vi "3D02_Grab_and_Attributes_Setup.vi"() -> ()   [LabVIEW 2012]
doc: "The Grab and Attributes Setup example VI allows the user to view the current attributes and settings, update attribute settings, acquire images continuously, and display the images in an image control."
uses:
  <vilib>/userDefined/High Color/IMAQdx.ctl
  <vilib>/vision/driver/IMAQdx.llb/IMAQdx Acquisition Mode.ctl
  <vilib>/vision/driver/IMAQdx.llb/IMAQdx Buffer Number Mode.ctl
  <vilib>/vision/driver/NI_Vision_Acquisition_Software.lvlib
  <resource>/objmgr/imaqdx.rc
  <userlib>/Photonfocus Toolkit/Photonfocus_Toolkit.lvlib
panel:
  out "MissedFrameCombineTriggerCounter":u8[](array[numeric])
  out "MissedBurstTriggerCounter":u8[](array[numeric])
  out "MissedTriggerCounter":u8[](array[numeric])
  out "EncoderPosition":u32[](array[numeric])
  out "RealTimeCounter":u32[](array[numeric])
  out "ImageCounter":u32[](array[numeric])
  out "Quality":u8[][](graph)
  out "Width":u8[][](graph)
  out "Peak":sgl[][](graph)
  out "FrameCombine_NrOfFrames":u32
  out "FrameCombine_Enable":bool
  out "PeakDetector_Mode":u32
  in  "Grab":bool
  out "Tooltip":string
  out "Units":string
  out "Tab Control Ref":T1
  in  "Tab Control":T2(tab)
  in  "U32 Value Control":u32(slide) scale=4.0..4044.0
  in  "DBL Value Control":dbl(slide) min=1.0 max=1028.0 step=1.0 scale=1.0..1028.0
  in  "String Value Control":string
  in  "Enum Value Control":u32(ring) items=["Mode_2Donly", "Mode_2Dand3D", "Mode_3Donly"]
  in  "Boolean Value Control":bool=TRUE
  in  "Command Value Control":bool
  in  "Attribute Table":string(tree)
  out "Frame Rate":dbl(knob) scale=0.0..100.0 scale format="%.1f"
  out "Image":T3(plugin-control)
  out "Buffer Number":u32
  in  "Camera Name":T4
  in  "stop":bool
  # "3D Data"
  # "Status info"
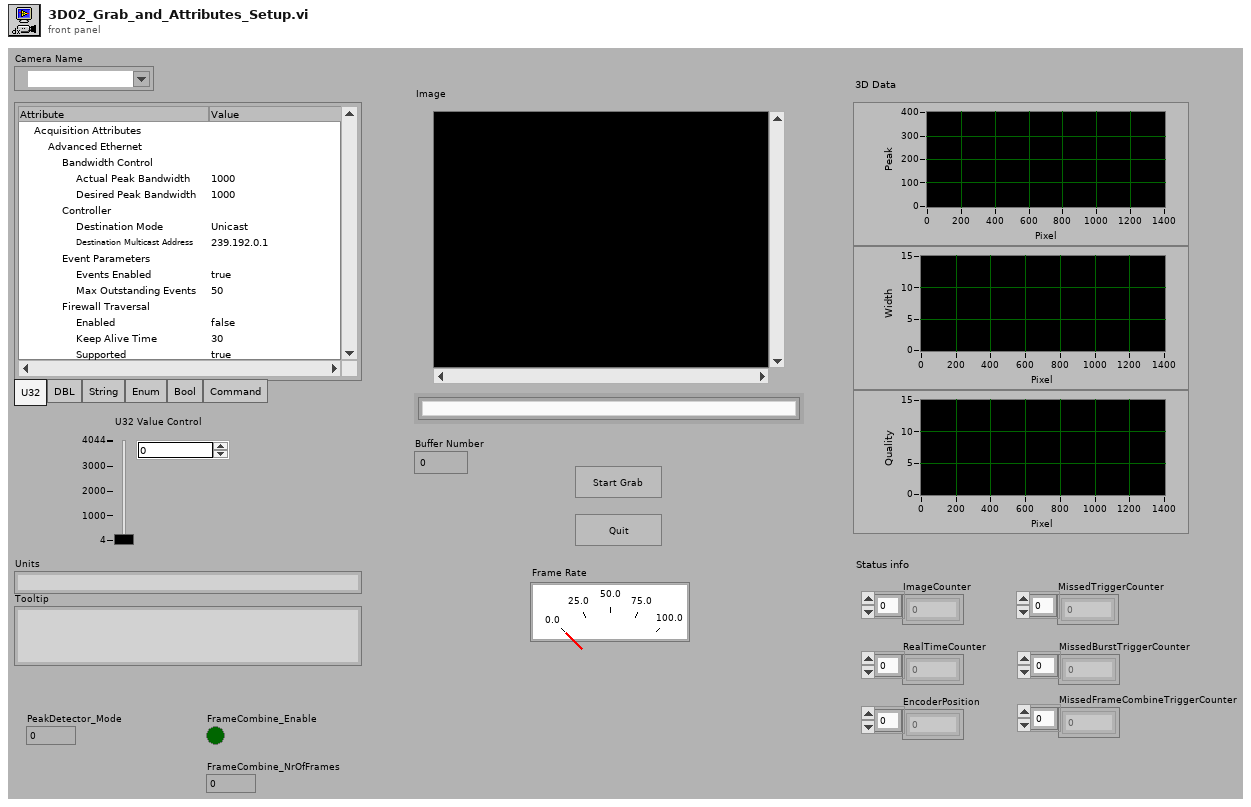
[diagram p1: front panel]
types:
  T1 = cluster{"Tab Control":refnum<vi>, "U32 Value Control":refnum<vi>, "DBL Value Control":refnum<vi>, "String Value Control":refnum<vi>, "Enum Value Control":refnum<vi>, "Boolean Value Control":refnum<vi>, "Command Value Control":refnum<vi>}
  T2 = enum32{"U32", "DBL", "String", "Enum", "Bool", "Command"}
  T3 = typedef "IMAQ Image.ctl" = refnum<image>
  T4 = typedef "IMAQdx.ctl" = refnum<k21>
  T5 = typedef "NI_Vision_Acquisition_Software.lvlib/IMAQdx Acquisition Mode.ctl" = enum32{"One Shot", "Continuous"}
  T6 = typedef "NI_Vision_Acquisition_Software.lvlib/IMAQdx Buffer Number Mode.ctl" = enum32{"Next", "Last", "Buffer Number"}
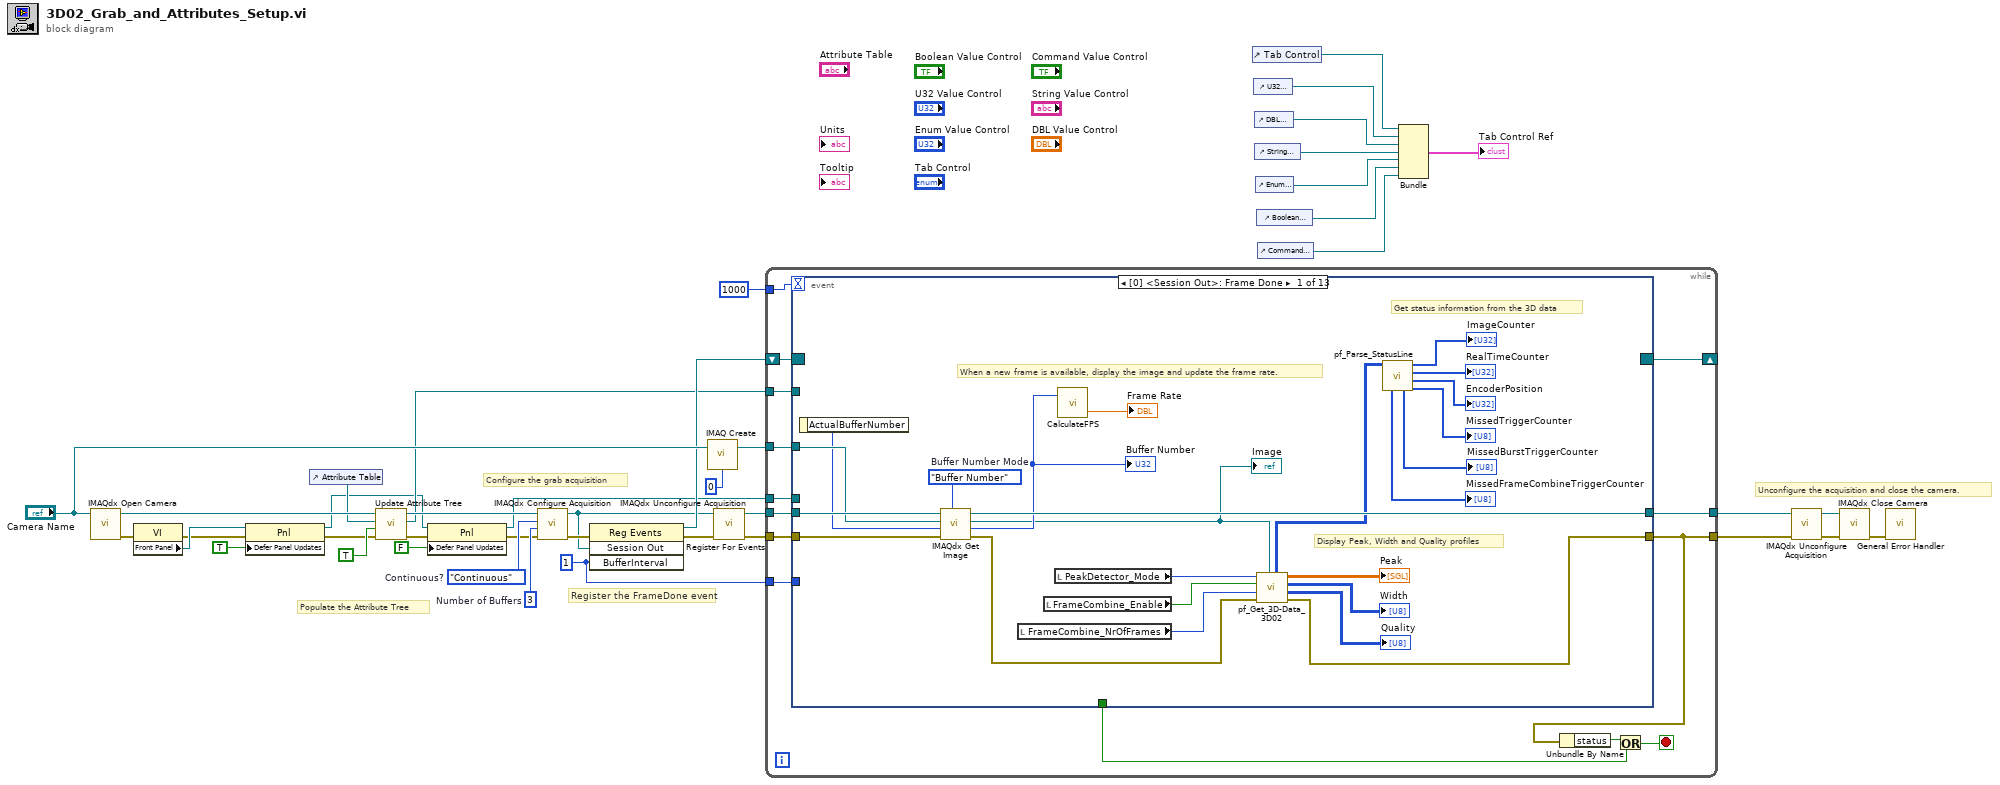
[diagram p0: block diagram]
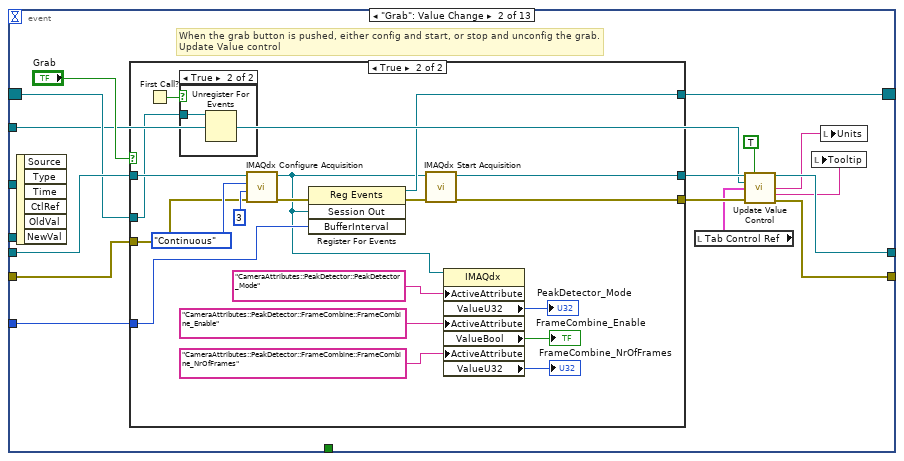
[diagram p2: hidden frame]
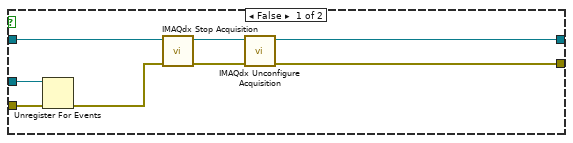
[diagram p3: hidden frame]
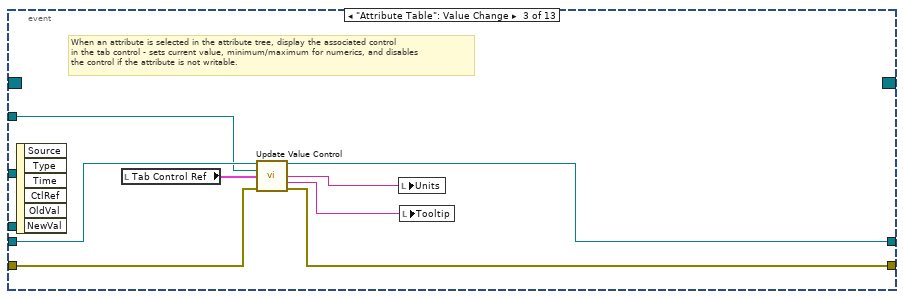
[diagram p5: hidden frame]
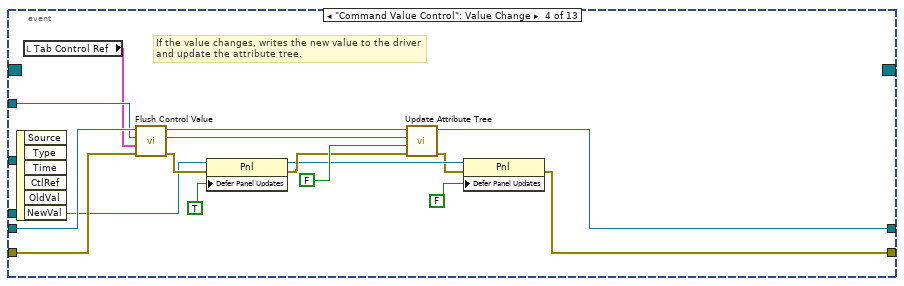
[diagram p6: hidden frame]
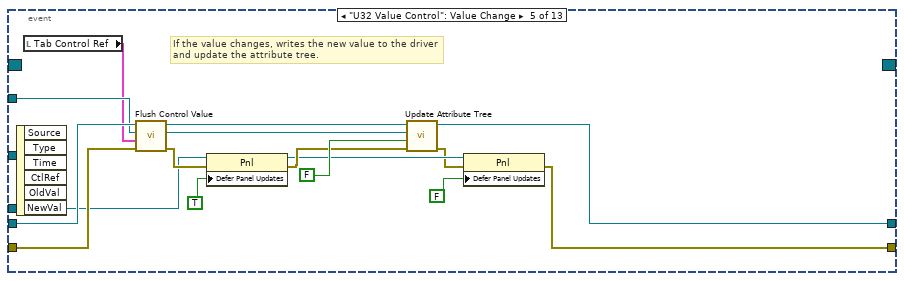
[diagram p7: hidden frame]
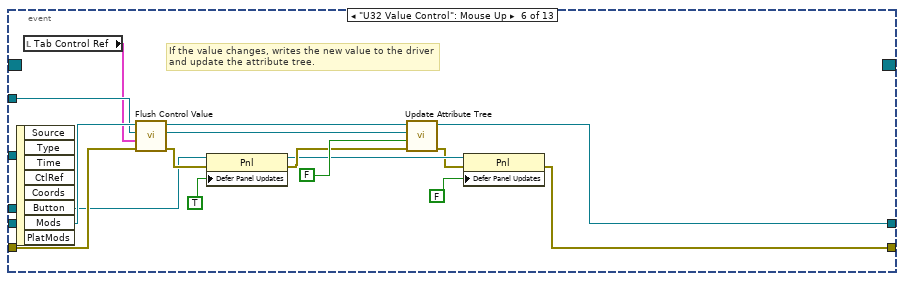
[diagram p8: hidden frame]
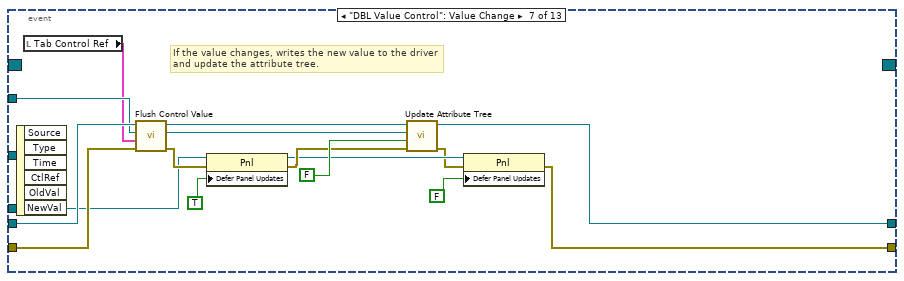
[diagram p9: hidden frame]
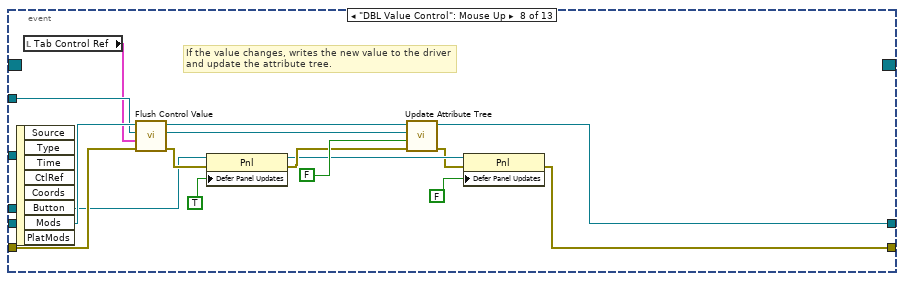
[diagram p10: hidden frame]
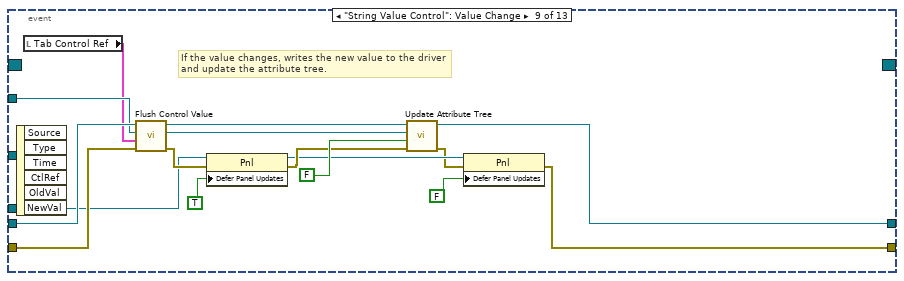
[diagram p11: hidden frame]
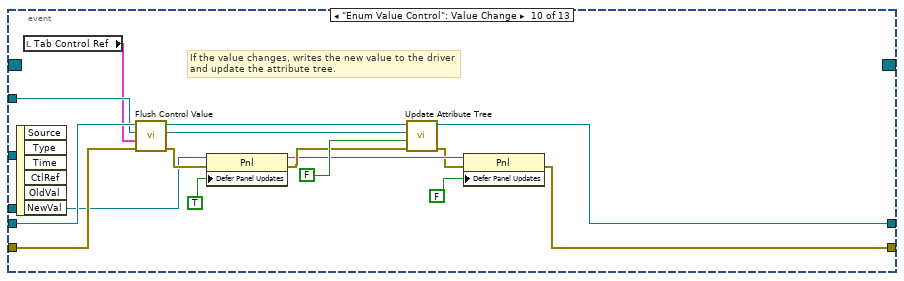
[diagram p12: hidden frame]
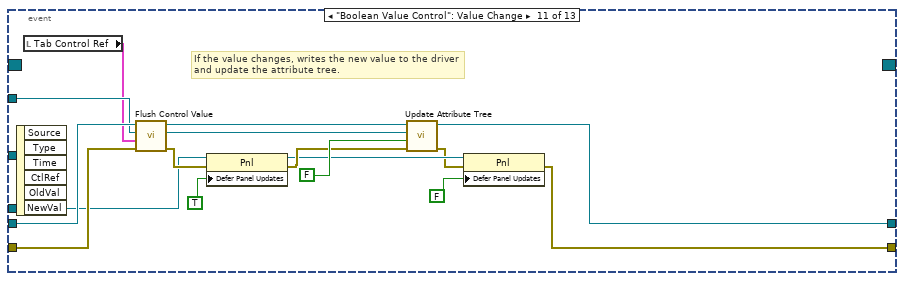
[diagram p13: hidden frame]
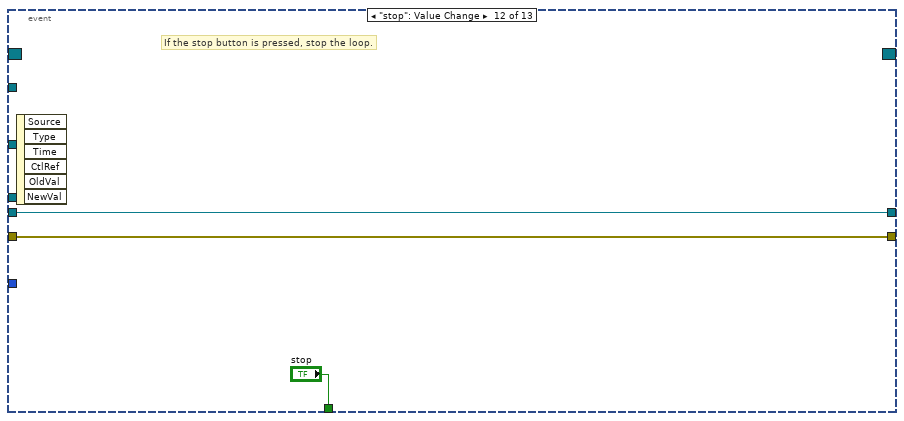
[diagram p14: hidden frame]
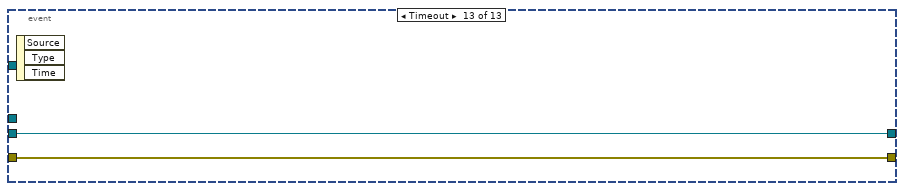
[diagram p15: hidden frame]
diagram:
  w6 = u32 1 ("BufferInterval")
  w37 = u32 3  # Number of Buffers
  w38 = IMAQdx_Acquisition_Mode."Continuous"  # Continuous?
  # "Unconfigure the acquisition and close the camera."
  # "Register the FrameDone event"
  # "Configure the grab acquisition"
  # "Populate the Attribute Tree"
  n1 = call <vilib>:"IMAQdx Open Camera.vi"("Session In"="Camera Name") -> ("error out"=w9:errorcluster, "Session Out"=w23:T4)  [unwired: 2 in, 7 out]
  n2 = property class="VI"(error in=w9) -> (error out=w10:errorcluster, "Front Panel"=w11:refnum<vi>)  [unwired: 1 in, 1 out]
  n3 = property class="Pnl"(reference=w11, error in=w10, "Defer Panel Updates"=TRUE) -> (reference out=w14:refnum<vi>, error out=w18:errorcluster)
  n4 = control-ref of="Attribute Table"() -> (w21:refnum<vi>)
  n5 = call <userlib>:"Update Attribute Tree.vi"("error in"=w18, "Flush Tree?"=TRUE, "Tree Control In"=w21, "Camera Name In"=w23) -> ("error out"=w17:errorcluster, "Tree Control Out"=w19:refnum<vi>, "Session Out"=w22:T4)  [unwired: 1 out]
  n6 = property class="Pnl"(reference=w14, error in=w17, "Defer Panel Updates"=FALSE) -> (reference out=w13:refnum<vi>, error out=w15:errorcluster)
  n7 = call <vilib>:"IMAQdx Configure Acquisition.vi"("error in"=w15, "Number of Buffers"=w37, "Continuous?"=w38, "Session In"=w22) -> ("error out"=w34:errorcluster, "Session Out"=w3:T4)  [unwired: 6 out]
  n8 = register-events(error in=w34, w3, w6) -> (reference out=w33:refnum<event-registration>, error out=w5:errorcluster)  [unwired: 1 in]
  n9 = call "IMAQ Create"("Image Name"="Camera Name", "Image Type"=0) -> ("New Image"=w41:T3)  [unwired: 2 in, 2 out]
  n10 = call <vilib>:"IMAQdx Unconfigure Acquisition.vi"("error in"=w5, "Session In"=w3) -> ("error out"=w4:errorcluster, "Session Out"=w2:T4)  [unwired: 8 out]
  n11 = while {
    tunnel: [w50] -> w8
    tunnel: w4 -> [w52]
    tunnel: w2 -> [w53]
    tunnel: [w49] -> w7
    tunnel: w41 -> [w51]
    tunnel: 1000 -> [w47]
    tunnel: w19 -> [w46]
    tunnel: w13 -> [w45]
    tunnel: w6 -> [w43]
    shift-right: [w42] -> _
    shift-left: w33 -> [w48]
    stop <- w55 stop-if-true
    n12 = event shown="[0] <Session Out>: Frame Done" {
      selector: w48 -> [_ w91 _ _ _ _ _ _ _ _ _ _ _]
      dyn-events: [_ w92 _ _ _ _ _ _ _ _ _ _ _] -> w42
      timeout: w47 -> [_ _ _ _ _ _ _ _ _ _ _ _ _]
      tunnel: w53 -> [w79 w94 w130 w145 w161 w177 w193 w209 w225 w241 w257 w260 w262]
      tunnel: w52 -> [w78 w90 w128 w146 w162 w178 w194 w210 w226 w242 w258 w259 w263]
      tunnel: w51 -> [w77 _ _ _ _ _ _ _ _ _ _ _ _]
      tunnel: [w76 w88 w129 w131 w147 w163 w179 w195 w211 w227 w243 w260 w262] -> w50
      tunnel: [w68 w86 w127 w132 w148 w164 w180 w196 w212 w228 w244 w259 w263] -> w49
      tunnel: w46 -> [_ w84 w123 w143 w159 w175 w191 w207 w223 w239 w255 _ _]
      tunnel: w45 -> [_ _ _ w137 w153 w169 w185 w201 w217 w233 w249 _ _]
      tunnel: [_ _ _ _ _ _ _ _ _ _ _ "stop" _] -> w44
      tunnel: w43 -> [_ w80 _ _ _ _ _ _ _ _ _ _ _]
      event event #0x0 {
        w74 = IMAQdx_Buffer_Number_Mode."Buffer Number"  # Buffer Number Mode
        # "Get status information from the 3D data"
        # "Display Peak, Width and Quality profiles"
        # "When a new frame is available, display the image and update the frame rate."
        n13 = event-data() -> ("ActualBufferNumber"=w73:u32)  [unwired: 1 out]
        n14 = call <vilib>:"IMAQdx Get Image.vi"("Buffer Number Mode (Next)"=w74, "error in"=w78, "Buffer Number In"=w73, "Image In"=w77, "Session In"=w79) -> ("error out"=w69:errorcluster, "Buffer Number Out"=w72:u32, "Image Out"=w70:T3, "Session Out"=w76:T4)  [unwired: 3 out]
        "Image" <- w70
        "Buffer Number" <- w72
        n15 = local read "FrameCombine_NrOfFrames"() -> (w63:u32)
        n16 = local read "FrameCombine_Enable"() -> (w64:bool)
        n17 = local read "PeakDetector_Mode"() -> (w71:u32)
        n18 = call <userlib>:"CalculateFPS.vi"("buffer number"=w72) -> ("processed FPS"=→"Frame Rate":dbl)  [unwired: 2 out]
        n19 = call <userlib>:"pf_Get_3D-Data_3D02.vi"("Aquired Image"=w70, "error in (no error)"=w69, "FrameCombine_NrOfFrames"=w63, "FrameCombine_Enable"=w64, "PealDetector_Mode"=w71) -> ("error out"=w68:errorcluster, "Quality Profile"=→"Quality":u8[][], "Width Profile"=→"Width":u8[][], "Peak Profile"=→"Peak":sgl[][], "Status Line"=w56:u8[][])  [unwired: 2 in]
        n20 = call <userlib>:"pf_Parse_StatusLine.vi"("Status Line"=w56) -> ("MissedTriggerCounter"=→"MissedTriggerCounter":u8[], "EncoderPosition"=→"EncoderPosition":u32[], "RealTimeCounter"=→"RealTimeCounter":u32[], "ImageCounter"=→"ImageCounter":u32[], "MissedBurstTriggerCounter"=→"MissedBurstTriggerCounter":u8[], "MissedFrameCombineTriggerCounter"=→"MissedFrameCombineTriggerCounter":u8[])  [unwired: 5 in]
      }
      event "Grab": Value Change {
        # "When the grab button is pushed, either config and start, or stop and unconfig the grab.\nUpdate Value control"
        n21 = event-data() -> ()  [unwired: 7 out]
        n22 = case shown="True" "Grab" {
          tunnel: w94 -> [w102 w119]
          tunnel: [w99 w121] -> w89
          tunnel: [w98 w120] -> w87
          tunnel: [_ w114] -> w92
          tunnel: w80 -> [_ w110]
          tunnel: w91 -> [w97 w112]
          tunnel: w90 -> [w95 w113]
          frame False {
            n23 = Unregister For Events(event registration refnum=w97, error in=w95) -> (error out=w96:errorcluster)
            n24 = call <vilib>:"IMAQdx Stop Acquisition.vi"("error in"=w96, "Session In"=w102) -> ("error out"=w100:errorcluster, "Session Out"=w101:T4)  [unwired: 8 out]
            n25 = call <vilib>:"IMAQdx Unconfigure Acquisition.vi"("error in"=w100, "Session In"=w101) -> ("error out"=w98:errorcluster, "Session Out"=w99:T4)  [unwired: 8 out]
          }
          frame True {
            n26 = First Call?() -> (First Call?: T/F=w111:bool)
            n27 = case shown="True" w111 {
              tunnel: w112 -> [_ w122]
              frame False {
              }
              frame True {
                n28 = Unregister For Events(event registration refnum=w122) -> ()  [unwired: 1 in, 1 out]
              }
            }
            n29 = call <vilib>:"IMAQdx Configure Acquisition.vi"("error in"=w113, "Number of Buffers"=u32 3, "Continuous?"=IMAQdx_Acquisition_Mode."Continuous", "Session In"=w119) -> ("error out"=w116:errorcluster, "Session Out"=w104:T4)  [unwired: 6 out]
            n30 = register-events(error in=w116, w104, w110) -> (reference out=w114:refnum<event-registration>, error out=w115:errorcluster)  [unwired: 1 in]
            n31 = call <vilib>:"IMAQdx Start Acquisition.vi"("error in"=w115, "Session In"=w104) -> ("error out"=w120:errorcluster, "Session Out"=w121:T4)  [unwired: 8 out]
            n32 = property class="IMAQdx"(reference=w104, "ActiveAttribute"="CameraAttributes::PeakDetector::PeakDetector_Mode", "ActiveAttribute"="CameraAttributes::PeakDetector::FrameCombine::FrameCombine_Enable", "ActiveAttribute"="CameraAttributes::PeakDetector::FrameCombine::FrameCombine_NrOfFrames") -> ("ValueU32"=→"PeakDetector_Mode":u32, "ValueBool"=→"FrameCombine_Enable":bool, "ValueU32"=→"FrameCombine_NrOfFrames":u32)  [unwired: 1 in, 2 out]
          }
        }
        n33 = local read "Tab Control Ref"() -> (w85:T1)
        n34 = call <userlib>:"Update Value Control.vi"("Session In"=w89, "Force update?"=TRUE, "Tree Control In"=w84, "Tab Control Ref In"=w85, "error in (no error)"=w87) -> ("Session Out"=w88:T4, "Units"=w83:string, "Tooltip"=w82:string, "error out"=w86:errorcluster)  [unwired: 7 out]
        n35 = local write "Tooltip"(w82) -> ()
        n36 = local write "Units"(w83) -> ()
      }
      event "Attribute Table": Value Change {
        # "When an attribute is selected in the attribute tree, display the associated control\nin the tab control - sets current value, minimum/maximum for numerics, and disables\nthe control if the attribute is not writable."
        n37 = event-data() -> ()  [unwired: 7 out]
        n38 = local read "Tab Control Ref"() -> (w126:T1)
        n39 = call <userlib>:"Update Value Control.vi"("Session In"=w130, "Tree Control In"=w123, "Tab Control Ref In"=w126, "error in (no error)"=w128) -> ("Session Out"=w129:T4, "Units"=w125:string, "Tooltip"=w124:string, "error out"=w127:errorcluster)  [unwired: 1 in, 7 out]
        n40 = local write "Units"(w125) -> ()
        n41 = local write "Tooltip"(w124) -> ()
      }
      event "Command Value Control": Value Change {
        # "If the value changes, writes the new value to the driver\nand update the attribute tree."
        n42 = event-data() -> ()  [unwired: 7 out]
        n43 = local read "Tab Control Ref"() -> (w142:T1)
        n44 = call <userlib>:"Flush Control Value.vi"("error in (no error)"=w146, "Tab Control Ref In"=w142, "Tree Control In"=w143, "Session In"=w145) -> ("error out"=w138:errorcluster, "Tree Control Out"=w141:refnum<vi>, "Session Out"=w144:T4)  [unwired: 1 out]
        n45 = property class="Pnl"(reference=w137, error in=w138, "Defer Panel Updates"=TRUE) -> (reference out=w135:refnum<vi>, error out=w139:errorcluster)
        n46 = call <userlib>:"Update Attribute Tree.vi"("error in"=w139, "Flush Tree?"=FALSE, "Tree Control In"=w141, "Camera Name In"=w144) -> ("error out"=w134:errorcluster, "Session Out"=w131:T4)  [unwired: 2 out]
        n47 = property class="Pnl"(reference=w135, error in=w134, "Defer Panel Updates"=FALSE) -> (error out=w132:errorcluster)  [unwired: 1 out]
      }
      event "U32 Value Control": Value Change {
        # "If the value changes, writes the new value to the driver\nand update the attribute tree."
        n48 = event-data() -> ()  [unwired: 7 out]
        n49 = local read "Tab Control Ref"() -> (w158:T1)
        n50 = call <userlib>:"Flush Control Value.vi"("error in (no error)"=w162, "Tab Control Ref In"=w158, "Tree Control In"=w159, "Session In"=w161) -> ("error out"=w154:errorcluster, "Tree Control Out"=w157:refnum<vi>, "Session Out"=w160:T4)  [unwired: 1 out]
        n51 = property class="Pnl"(reference=w153, error in=w154, "Defer Panel Updates"=TRUE) -> (reference out=w151:refnum<vi>, error out=w155:errorcluster)
        n52 = call <userlib>:"Update Attribute Tree.vi"("error in"=w155, "Flush Tree?"=FALSE, "Tree Control In"=w157, "Camera Name In"=w160) -> ("error out"=w150:errorcluster, "Session Out"=w147:T4)  [unwired: 2 out]
        n53 = property class="Pnl"(reference=w151, error in=w150, "Defer Panel Updates"=FALSE) -> (error out=w148:errorcluster)  [unwired: 1 out]
      }
      event "U32 Value Control": Mouse Up {
        # "If the value changes, writes the new value to the driver\nand update the attribute tree."
        n54 = event-data() -> ()  [unwired: 9 out]
        n55 = local read "Tab Control Ref"() -> (w174:T1)
        n56 = call <userlib>:"Flush Control Value.vi"("error in (no error)"=w178, "Tab Control Ref In"=w174, "Tree Control In"=w175, "Session In"=w177) -> ("error out"=w170:errorcluster, "Tree Control Out"=w173:refnum<vi>, "Session Out"=w176:T4)  [unwired: 1 out]
        n57 = property class="Pnl"(reference=w169, error in=w170, "Defer Panel Updates"=TRUE) -> (reference out=w167:refnum<vi>, error out=w171:errorcluster)
        n58 = call <userlib>:"Update Attribute Tree.vi"("error in"=w171, "Flush Tree?"=FALSE, "Tree Control In"=w173, "Camera Name In"=w176) -> ("error out"=w166:errorcluster, "Session Out"=w163:T4)  [unwired: 2 out]
        n59 = property class="Pnl"(reference=w167, error in=w166, "Defer Panel Updates"=FALSE) -> (error out=w164:errorcluster)  [unwired: 1 out]
      }
      event "DBL Value Control": Value Change {
        # "If the value changes, writes the new value to the driver\nand update the attribute tree."
        n60 = event-data() -> ()  [unwired: 7 out]
        n61 = local read "Tab Control Ref"() -> (w190:T1)
        n62 = call <userlib>:"Flush Control Value.vi"("error in (no error)"=w194, "Tab Control Ref In"=w190, "Tree Control In"=w191, "Session In"=w193) -> ("error out"=w186:errorcluster, "Tree Control Out"=w189:refnum<vi>, "Session Out"=w192:T4)  [unwired: 1 out]
        n63 = property class="Pnl"(reference=w185, error in=w186, "Defer Panel Updates"=TRUE) -> (reference out=w183:refnum<vi>, error out=w187:errorcluster)
        n64 = call <userlib>:"Update Attribute Tree.vi"("error in"=w187, "Flush Tree?"=FALSE, "Tree Control In"=w189, "Camera Name In"=w192) -> ("error out"=w182:errorcluster, "Session Out"=w179:T4)  [unwired: 2 out]
        n65 = property class="Pnl"(reference=w183, error in=w182, "Defer Panel Updates"=FALSE) -> (error out=w180:errorcluster)  [unwired: 1 out]
      }
      event "DBL Value Control": Mouse Up {
        # "If the value changes, writes the new value to the driver\nand update the attribute tree."
        n66 = event-data() -> ()  [unwired: 9 out]
        n67 = local read "Tab Control Ref"() -> (w206:T1)
        n68 = call <userlib>:"Flush Control Value.vi"("error in (no error)"=w210, "Tab Control Ref In"=w206, "Tree Control In"=w207, "Session In"=w209) -> ("error out"=w202:errorcluster, "Tree Control Out"=w205:refnum<vi>, "Session Out"=w208:T4)  [unwired: 1 out]
        n69 = property class="Pnl"(reference=w201, error in=w202, "Defer Panel Updates"=TRUE) -> (reference out=w199:refnum<vi>, error out=w203:errorcluster)
        n70 = call <userlib>:"Update Attribute Tree.vi"("error in"=w203, "Flush Tree?"=FALSE, "Tree Control In"=w205, "Camera Name In"=w208) -> ("error out"=w198:errorcluster, "Session Out"=w195:T4)  [unwired: 2 out]
        n71 = property class="Pnl"(reference=w199, error in=w198, "Defer Panel Updates"=FALSE) -> (error out=w196:errorcluster)  [unwired: 1 out]
      }
      event "String Value Control": Value Change {
        # "If the value changes, writes the new value to the driver\nand update the attribute tree."
        n72 = event-data() -> ()  [unwired: 7 out]
        n73 = local read "Tab Control Ref"() -> (w222:T1)
        n74 = call <userlib>:"Flush Control Value.vi"("error in (no error)"=w226, "Tab Control Ref In"=w222, "Tree Control In"=w223, "Session In"=w225) -> ("error out"=w218:errorcluster, "Tree Control Out"=w221:refnum<vi>, "Session Out"=w224:T4)  [unwired: 1 out]
        n75 = property class="Pnl"(reference=w217, error in=w218, "Defer Panel Updates"=TRUE) -> (reference out=w215:refnum<vi>, error out=w219:errorcluster)
        n76 = call <userlib>:"Update Attribute Tree.vi"("error in"=w219, "Flush Tree?"=FALSE, "Tree Control In"=w221, "Camera Name In"=w224) -> ("error out"=w214:errorcluster, "Session Out"=w211:T4)  [unwired: 2 out]
        n77 = property class="Pnl"(reference=w215, error in=w214, "Defer Panel Updates"=FALSE) -> (error out=w212:errorcluster)  [unwired: 1 out]
      }
      event "Enum Value Control": Value Change {
        # "If the value changes, writes the new value to the driver\nand update the attribute tree."
        n78 = event-data() -> ()  [unwired: 7 out]
        n79 = local read "Tab Control Ref"() -> (w238:T1)
        n80 = call <userlib>:"Flush Control Value.vi"("error in (no error)"=w242, "Tab Control Ref In"=w238, "Tree Control In"=w239, "Session In"=w241) -> ("error out"=w234:errorcluster, "Tree Control Out"=w237:refnum<vi>, "Session Out"=w240:T4)  [unwired: 1 out]
        n81 = property class="Pnl"(reference=w233, error in=w234, "Defer Panel Updates"=TRUE) -> (reference out=w231:refnum<vi>, error out=w235:errorcluster)
        n82 = call <userlib>:"Update Attribute Tree.vi"("error in"=w235, "Flush Tree?"=FALSE, "Tree Control In"=w237, "Camera Name In"=w240) -> ("error out"=w230:errorcluster, "Session Out"=w227:T4)  [unwired: 2 out]
        n83 = property class="Pnl"(reference=w231, error in=w230, "Defer Panel Updates"=FALSE) -> (error out=w228:errorcluster)  [unwired: 1 out]
      }
      event "Boolean Value Control": Value Change {
        # "If the value changes, writes the new value to the driver\nand update the attribute tree."
        n84 = event-data() -> ()  [unwired: 7 out]
        n85 = local read "Tab Control Ref"() -> (w254:T1)
        n86 = call <userlib>:"Flush Control Value.vi"("error in (no error)"=w258, "Tab Control Ref In"=w254, "Tree Control In"=w255, "Session In"=w257) -> ("error out"=w250:errorcluster, "Tree Control Out"=w253:refnum<vi>, "Session Out"=w256:T4)  [unwired: 1 out]
        n87 = property class="Pnl"(reference=w249, error in=w250, "Defer Panel Updates"=TRUE) -> (reference out=w247:refnum<vi>, error out=w251:errorcluster)
        n88 = call <userlib>:"Update Attribute Tree.vi"("error in"=w251, "Flush Tree?"=FALSE, "Tree Control In"=w253, "Camera Name In"=w256) -> ("error out"=w246:errorcluster, "Session Out"=w243:T4)  [unwired: 2 out]
        n89 = property class="Pnl"(reference=w247, error in=w246, "Defer Panel Updates"=FALSE) -> (error out=w244:errorcluster)  [unwired: 1 out]
      }
      event "stop": Value Change {
        # "If the stop button is pressed, stop the loop."
        n90 = event-data() -> ()  [unwired: 7 out]
      }
      event Timeout {
        n91 = event-data() -> ()  [unwired: 4 out]
      }
    }
    n92 = Unbundle By Name(w49) -> ("status"=w54:bool)
    n93 = Or(x=w54, y=w44) -> (x .or. y?=w55:bool)
  }
  n94 = control-ref of="Tab Control"() -> (w31:refnum<vi>)
  n95 = control-ref of="U32 Value Control"() -> (w29:refnum<vi>)
  n96 = control-ref of="DBL Value Control"() -> (w28:refnum<vi>)
  n97 = control-ref of="String Value Control"() -> (w30:refnum<vi>)
  n98 = control-ref of="Enum Value Control"() -> (w27:refnum<vi>)
  n99 = control-ref of="Boolean Value Control"() -> (w26:refnum<vi>)
  n100 = control-ref of="Command Value Control"() -> (w25:refnum<vi>)
  n101 = Bundle("Tab Control"=w31, "U32 Value Control"=w29, "DBL Value Control"=w28, "String Value Control"=w30, "Enum Value Control"=w27, "Boolean Value Control"=w26, "Command Value Control"=w25) -> (→"Tab Control Ref":T1)  [unwired: 1 out]
  n102 = call <vilib>:"IMAQdx Unconfigure Acquisition.vi"("error in"=w7, "Session In"=w8) -> ("error out"=w36:errorcluster, "Session Out"=w35:T4)  [unwired: 8 out]
  n103 = call <vilib>:"IMAQdx Close Camera.vi"("error in"=w36, "Session In"=w35) -> ("error out"=w40:errorcluster)  [unwired: 9 out]
  n104 = call <vilib>:"General Error Handler.vi"("error in (no error)"=w40) -> ()  [unwired: 1 in, 14 out]
